vi "Edges position.vi"(10 "Detected Objects":T1[](array[typedef]) {"Bounding Box"."y" format="%.2f"; "Bounding Box"."x" format="%.2f"}, 11 "Minimum Score Threshold":sgl) -> (0 "bottom border":sgl, 1 "left border":sgl, 2 "right border":sgl, 3 "Cars found":i32, 5 "Car found":bool, 7 "nearest car object":T1[](array[typedef]) {"Bounding Box"."y" format="%.2f"; "Bounding Box"."x" format="%.2f"})   [LabVIEW 2020]
uses:
  <vilib>/vision/Deep Learning.llb/IMAQ DL Model Objects.ctl
panel:
  in  "reset center values":bool
  out "distance":dbl(graph)
  in  "distance threshold":dbl=100.0
  out "top border":sgl
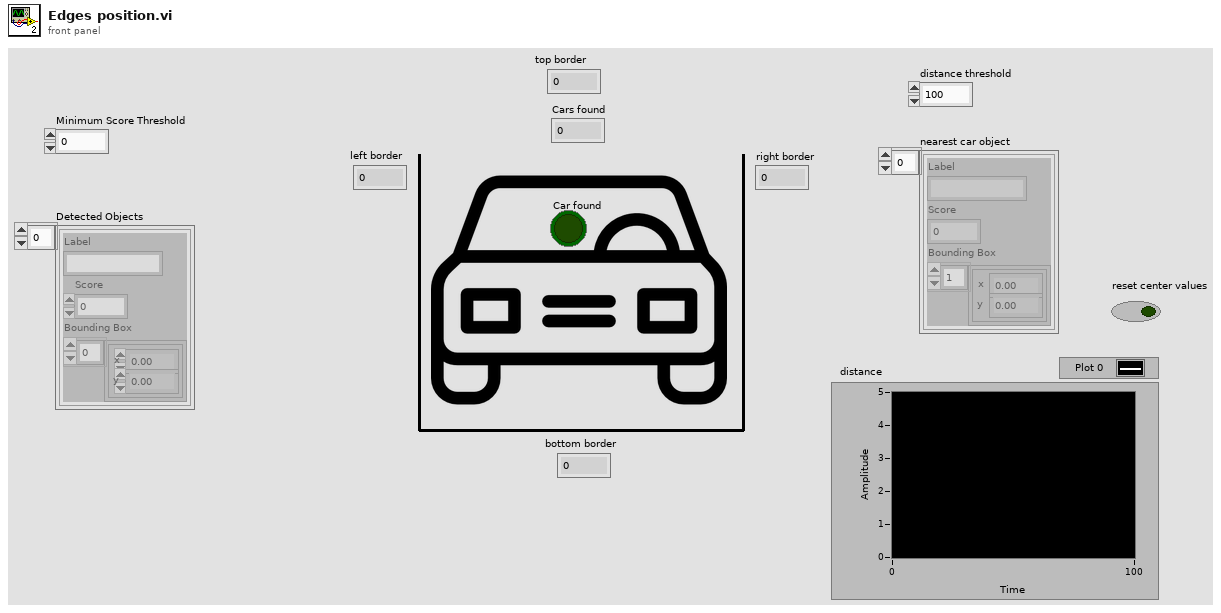
[diagram p1: front panel]
types:
  T1 = typedef "IMAQ DL Model Objects.ctl" = cluster{"Label":string, "Score":sgl, "Bounding Box":cluster{"x":sgl, "y":sgl}[]}
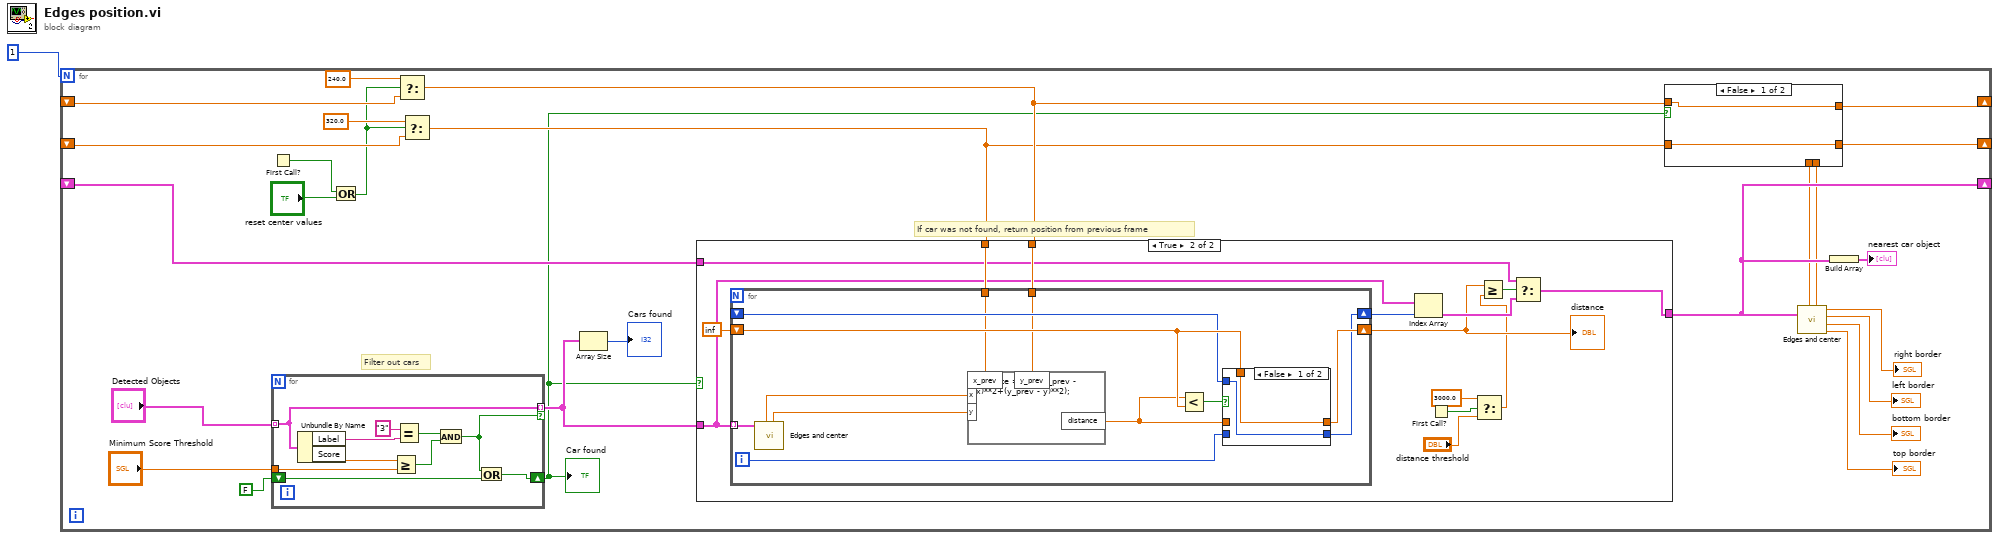
[diagram p0: block diagram]
diagram:
  n1 = for {
    N: 1 -> [_]
    shift-right: [w23] -> _
    shift-left: _ -> [w13]
    shift-right: [w24] -> _
    shift-left: _ -> [w11]
    shift-right: [w16] -> _
    shift-left: _ -> [w18]
    # "Filter out cars"
    # "If car was not found, return position from previous frame"
    n2 = First Call?() -> (First Call?: T/F=w3:bool)
    n3 = for {
      tunnel: "Detected Objects" -> [w72] mode=indexing
      tunnel: [w72] -> w19 mode=indexing if=w66
      tunnel: "Minimum Score Threshold" -> [w69]
      shift-right: [w68] -> w5
      shift-left: FALSE -> [w67]
      n4 = Unbundle By Name(w72) -> ("Label"=w65:string, "Score"=w71:sgl)
      n5 = Greater Or Equal?(x=w71, y=w69) -> (x >= y?=w64:bool)
      n6 = Equal?(x="3", y=w65) -> (x = y?=w63:bool)
      n7 = And(x=w63, y=w64) -> (x .and. y?=w66:bool)
      n8 = Or(x=w66, y=w67) -> (x .or. y?=w68:bool)
    }
    "Car found" <- w5
    n9 = Or(x=w3, y="reset center values") -> (x .or. y?=w2:bool)
    n10 = Select(t=sgl 240.0 ("y"), s=w2, f=w13) -> (s? t:f=w14:sgl)
    n11 = Select(t=sgl 320.0 ("y"), s=w2, f=w11) -> (s? t:f=w10:sgl)
    n12 = Array Size(array=w19) -> (size(s)=→"Cars found":i32)
    n13 = case shown="True" w5 {
      tunnel: w19 -> [_ w42]
      tunnel: [w32 w39] -> w16
      tunnel: w10 -> [_ w45]
      tunnel: w14 -> [_ w44]
      tunnel: w18 -> [w32 w38]
      frame False {
      }
      frame True {
        n14 = for {
          tunnel: w42 -> [w49] mode=indexing
          shift-right: [w58] -> w37
          shift-left: inf -> [w55]
          shift-right: [w56] -> w43
          shift-left: _ -> [w53]
          tunnel: w45 -> [w50]
          tunnel: w44 -> [w51]
          i -> [w57]
          n15 = call "Edges and center.vi"("Class Result"=w49) -> ("y center"=w47:sgl, "x center"=w48:sgl)  [unwired: 5 in, 4 out]
          n16 = formula code="distance = sqrt((x_prev - x)**2+(y_prev - y)**2);"("x"=w48, "y"=w47, "x_prev"=w50, "y_prev"=w51) -> ("distance"=w52:dbl)
          n17 = Less?(x=w52, y=w55) -> (x < y?=w54:bool)
          n18 = case shown="False" w54 {
            tunnel: w52 -> [_ w62]
            tunnel: [w60 w62] -> w58
            tunnel: w55 -> [w60 _]
            tunnel: w57 -> [_ w61]
            tunnel: [w59 w61] -> w56
            tunnel: w53 -> [w59 _]
            frame False {
            }
            frame True {
            }
          }
        }
        "distance" <- w37
        n19 = Index Array(array=w42, index=w43) -> (element=w40:T1)
        n20 = First Call?() -> (First Call?: T/F=w36:bool)
        n21 = Select(t=3000.0, s=w36, f="distance threshold") -> (s? t:f=w33:dbl)
        n22 = Greater Or Equal?(x=w37, y=w33) -> (x >= y?=w41:bool)
        n23 = Select(t=w38, s=w41, f=w40) -> (s? t:f=w39:T1)
      }
    }
    n24 = call "Edges and center.vi"("Class Result"=w16) -> ("y2"=→"top border":sgl, "y"=→"bottom border":sgl, "x2"=→"left border":sgl, "x"=→"right border":sgl, "y center"=w6:sgl, "x center"=w7:sgl)  [unwired: 5 in]
    n25 = case shown="False" w5 {
      tunnel: w10 -> [w29 _]
      tunnel: [w29 w31] -> w24
      tunnel: w7 -> [_ w31]
      tunnel: w6 -> [_ w30]
      tunnel: [w28 w30] -> w23
      tunnel: w14 -> [w28 _]
      frame False {
      }
      frame True {
      }
    }
    n26 = Build Array(w16) -> (→"nearest car object":T1[])
  }
